vi "Update messages.vi"(8 "error in (no error)":errorcluster, 11 "Header content in":refnum<class "Header content.lvclass">) -> (0 "error out":errorcluster, 3 "Header content out":refnum<class "Header content.lvclass">)   [LabVIEW 2018, in "Header content.lvclass"]
uses:
  Header content.lvclass
  Header content.lvclass/Header content.ctl
  RxTx/RxTx.lvclass
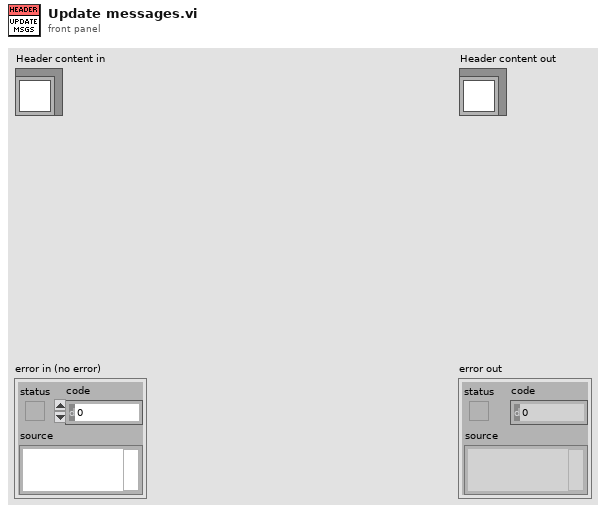
[diagram p1: front panel]
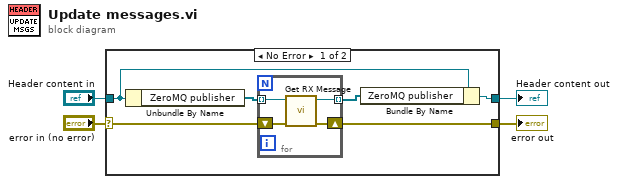
[diagram p0: block diagram]
diagram:
  n1 = case shown="No Error" "error in (no error)" {
    selector: "error in (no error)" -> [w10 w16]
    tunnel: [w9 w16] -> w3
    tunnel: [w7 w15] -> w1
    tunnel: "Header content in" -> [w8 w15]
    frame No Error {
      n2 = Unbundle By Name(w8) -> ("ZeroMQ publisher"=w5:refnum<class "RxTx.lvclass">[])
      n3 = for {
        shift-right: [w13] -> w9
        shift-left: w10 -> [w14]
        tunnel: [w12] -> w6 mode=indexing
        tunnel: w5 -> [w11] mode=indexing
        n4 = call "Get RX Message.vi"("error in (no error)"=w14, "RxTx in"=w11) -> ("error out"=w13:errorcluster, "RxTx out"=w12:refnum<class "RxTx.lvclass">)  [unwired: 8 in]
      }
      n5 = Bundle By Name(cluster=w8, "ZeroMQ publisher"=w6) -> (w7:refnum<class "Header content.lvclass">)
    }
    frame Error {
    }
  }
  "error out" <- w3
  "Header content out" <- w1
